vi "Test_WriteValue_InvalidRefnum_Error.vi"(8 "error in (no error)":errorcluster, 11 "TestCase in":refnum<class "TestListboxItemNamesBinding.lvclass">) -> (0 "error out":errorcluster, 3 "TestCase out":refnum<class "TestListboxItemNamesBinding.lvclass">)   [LabVIEW 2017, in "TestListboxItemNamesBinding.lvclass"]
uses:
  TestListboxItemNamesBinding.lvclass
  Source/Concrete/ListboxItemNamesBinding/ListboxItemNamesBinding.lvclass/ListboxItemNamesBinding.ctl
  Source/Concrete/ListboxItemNamesBinding/ListboxItemNamesBinding.lvclass
  C:/Git/composed-transport/Source/ITransport/ITransport.lvclass
  <vilib>/Utility/error.llb/Error Cluster From Error Code.vi
  Source/ITransport/ITransport.lvclass
panel:
  out "Return Error":errorcluster
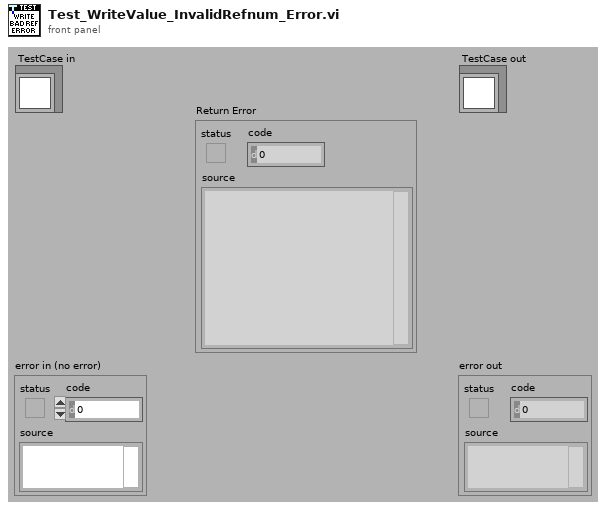
[diagram p1: front panel]
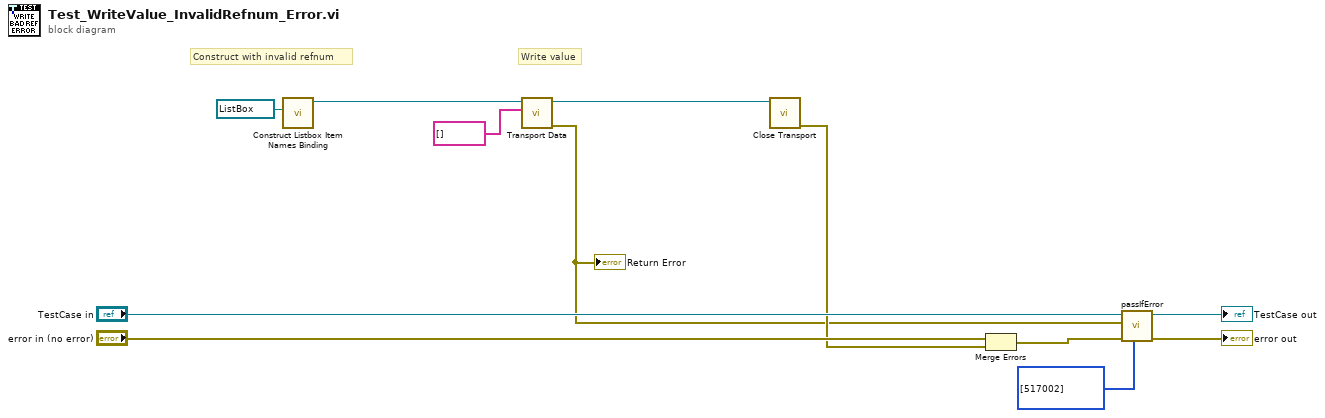
[diagram p0: block diagram]
diagram:
  # "Construct with invalid refnum"
  # "Write value"
  n1 = call "Construct Listbox Item Names Binding.vi"("LstBox Refnum"=refnum<vi> refnum) -> ("ListboxItemNamesBinding"=w8:refnum<class "ListboxItemNamesBinding.lvclass">)  [unwired: 9 in, 1 out]
  n2 = call "Transport Data.vi"("Value"=string[] [] ("Format String"), "ITransport in"=w8) -> ("error out"=w3:errorcluster, "ITransport out"=w6:refnum<class "ListboxItemNamesBinding.lvclass">)  [unwired: 8 in]
  "Return Error" <- w3
  n3 = call-dynamic "Close Transport.vi"("ITransport in"=w6) -> ("error out"=w5:errorcluster)  [unwired: 10 in]
  n4 = Merge Errors("error in (no error)", w5) -> (w7:errorcluster)
  n5 = call-dynamic "passIfError.vi"("passing error codes (default = any error code)"=i32[] [517002], "error in (no error)"=w7, "error"=w3, "TestCase in"="TestCase in") -> ("error out"=→"error out":errorcluster, "TestCase out"=→"TestCase out":refnum<class "TestListboxItemNamesBinding.lvclass">)  [unwired: 6 in]
